vi "Reset.vi"(8 "error in (no error)":errorcluster, 9 "Delay After Reset (2000 ms)":u32=2000, 10 "Motor ID (0)":u8, 11 "Dynamixel Motor VISA in":refnum<class "Dynamixel Motor VISA.lvclass">) -> (0 "error out":errorcluster, 3 "Dynamixel Motor VISA out":refnum<class "Dynamixel Motor VISA.lvclass">)   [LabVIEW 2016, in "Dynamixel Motor VISA.lvclass"]
doc: "Resets the motor and to its default values. The motor ID will be 1 and the baud rate will be 57600 bps."
uses:
  <instrlib>/Dynamixel Motor/HAIOL/VISA/Dynamixel Motor VISA.lvclass
  <instrlib>/Dynamixel Motor/HAIOL/VISA/Dynamixel Motor VISA.lvclass/Dynamixel Motor VISA.ctl
  <instrlib>/Dynamixel Motor/Dynamixel Motor.lvlib
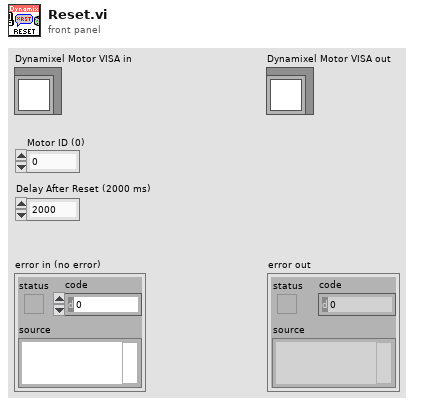
[diagram p1: front panel]
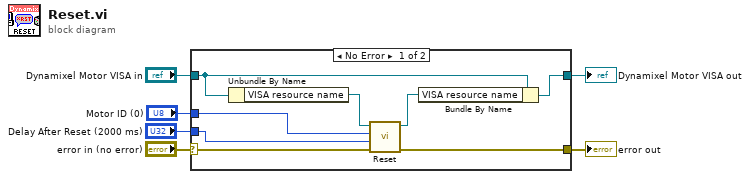
[diagram p0: block diagram]
diagram:
  n1 = case shown="No Error" "error in (no error)" {
    selector: "error in (no error)" -> [w14 w15]
    tunnel: "Dynamixel Motor VISA in" -> [w8 w16]
    tunnel: "Motor ID (0)" -> [w12 _]
    tunnel: "Delay After Reset (2000 ms)" -> [w11 _]
    tunnel: [w10 w15] -> w2
    tunnel: [w7 w16] -> w1
    frame No Error {
      n2 = Unbundle By Name(w8) -> ("VISA resource name"=w13:refnum<visa-resource-name>)
      n3 = call <instrlib>:"Reset.vi"("Error In (no error)"=w14, "Delay After Reset (2000 ms)"=w11, "Motor ID (0)"=w12, "VISA resource name"=w13) -> ("error out"=w10:errorcluster, "VISA resource name out"=w9:refnum<visa-resource-name>)  [unwired: 6 in]
      n4 = Bundle By Name(cluster=w8, "VISA resource name"=w9) -> (w7:refnum<class "Dynamixel Motor VISA.lvclass">)
    }
    frame Error {
    }
  }
  "error out" <- w2
  "Dynamixel Motor VISA out" <- w1
